vi "save_dim3_array.vi"(8 "error in (no error)":errorcluster, 10 "ana/scan data array":T1, 11 "DataLogging in":refnum<class "DataLogging.lvclass">) -> (0 "error out":errorcluster, 3 "DataLogging out":refnum<class "DataLogging.lvclass">)   [LabVIEW 2017, in "DataLogging.lvclass"]
doc: "The input array (dim3) is being saved into the datafile/database.\nThe datalog object stores the path of the logfile and other\nparameters for each analysis"
uses:
  DataLogging.lvclass
  Analysis/AnalysisDataArray.ctl
  ValueArray.ctl
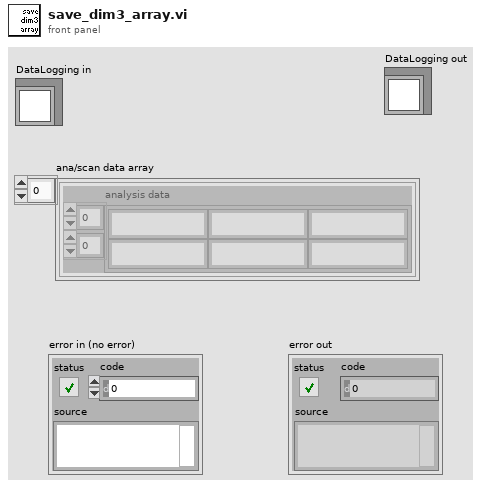
[diagram p1: front panel]
types:
  T1 = typedef "AnalysisDataArray.ctl" = cluster{"analysis data":string[][]}[]
  T2 = typedef "ValueArray.ctl" = string[]
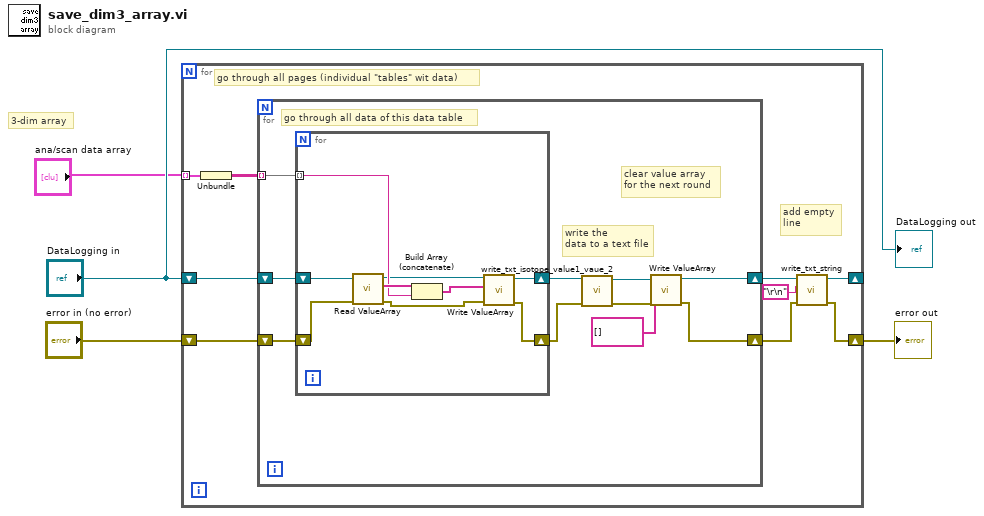
[diagram p0: block diagram]
diagram:
  # "3-dim array"
  n1 = for {
    tunnel: "ana/scan data array" -> [w5] mode=indexing
    shift-right: [w8] -> w3
    shift-left: "error in (no error)" -> [w12]
    shift-right: [w7] -> _
    shift-left: "DataLogging in" -> [w13]
    # "add empty\nline"
    # "go through all pages (individual \"tables\" wit data)"
    n2 = Unbundle(w5) -> ("analysis data"=w6:string[][])
    n3 = for {
      tunnel: w6 -> [w23] mode=indexing
      shift-right: [w15] -> w9
      shift-left: w12 -> [w21]
      shift-right: [w16] -> w11
      shift-left: w13 -> [w22]
      # "clear value array\nfor the next round"
      # "write the\ndata to a text file"
      # "go through all data of this data table"
      n4 = for {
        tunnel: w23 -> [w29] mode=indexing
        shift-right: [w25] -> w20
        shift-left: w22 -> [w32]
        shift-right: [w24] -> w19
        shift-left: w21 -> [w31]
        n5 = call-dynamic "Read ValueArray.vi"("error in (no error)"=w31, "DataLogging in"=w32) -> ("error out"=w26:errorcluster, "ValueArray"=w30:T2, "DataLogging out"=w27:refnum<class "DataLogging.lvclass">)  [unwired: 7 in]
        n6 = Build Array (concatenate)(w30, w29) -> (w28:T2)
        n7 = call-dynamic "Write ValueArray.vi"("error in (no error)"=w26, "ValueArray"=w28, "DataLogging in"=w27) -> ("error out"=w24:errorcluster, "DataLogging out"=w25:refnum<class "DataLogging.lvclass">)  [unwired: 7 in]
      }
      n8 = call-dynamic "write_txt_isotope_value1_vaue_2.vi"("error in (no error)"=w19, "DataLoggingText in"=w20) -> ("error out"=w17:errorcluster, "DataLoggingText out"=w18:refnum<class "DataLogging.lvclass">)  [unwired: 8 in]
      n9 = call-dynamic "Write ValueArray.vi"("error in (no error)"=w17, "ValueArray"=T2 [], "DataLogging in"=w18) -> ("error out"=w15:errorcluster, "DataLogging out"=w16:refnum<class "DataLogging.lvclass">)  [unwired: 7 in]
    }
    n10 = call-dynamic "write_txt_string.vi"("error in (no error)"=w9, "data string"="\r\n", "DataLoggingText in"=w11) -> ("error out"=w8:errorcluster, "DataLoggingText out"=w7:refnum<class "DataLogging.lvclass">)  [unwired: 7 in]
  }
  "error out" <- w3
  "DataLogging out" <- "DataLogging in"
